vi "Read Data.vi"(8 "error in (no error)":errorcluster, 11 "U16 in":refnum<class "U16.lvclass">) -> (0 "error out":errorcluster, 2 "Data":u16, 3 "U16 out":refnum<class "U16.lvclass">)   [LabVIEW 2014, in "Base Data Class.lvlib" / "U16.lvclass"]
uses:
  U16.lvclass
  U16.lvclass/U16.ctl
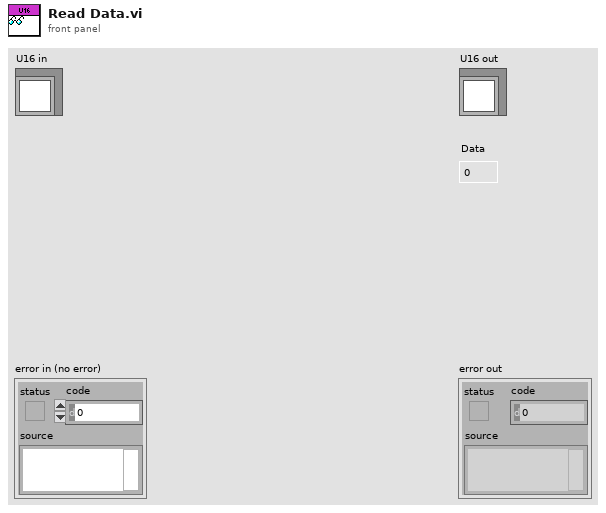
[diagram p1: front panel]
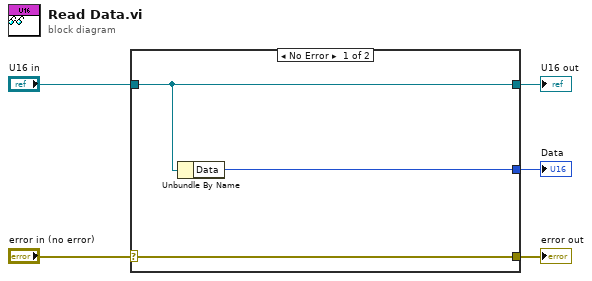
[diagram p0: block diagram]
diagram:
  n1 = case shown="No Error" "error in (no error)" {
    selector: "error in (no error)" -> [w8 w9]
    tunnel: [w8 w9] -> w4
    tunnel: [w7 w10] -> w2
    tunnel: "U16 in" -> [w7 w10]
    tunnel: [w6 _] -> w1
    frame No Error {
      n2 = Unbundle By Name(w7) -> ("Data"=w6:u16)
    }
    frame Error {
    }
  }
  "error out" <- w4
  "U16 out" <- w2
  "Data" <- w1
